vi "DisplayText.vi"(10 "text":string, 11 "Grid":T1) -> (3 "new picture":picture)   [LabVIEW 2020]
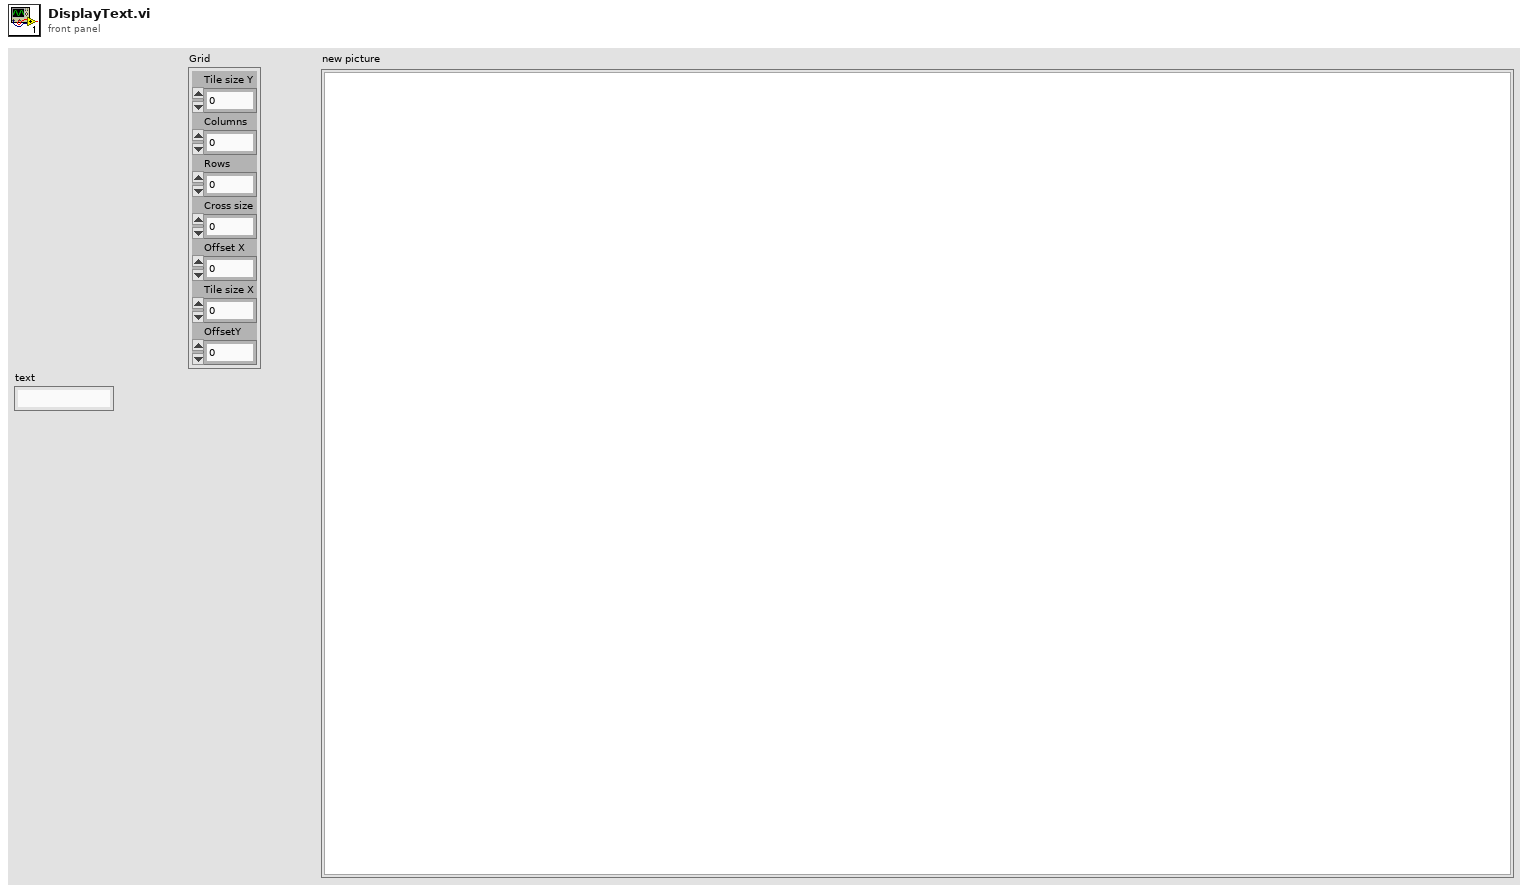
[diagram p1: front panel]
types:
  T1 = cluster{"Tile size Y":dbl, "Columns":dbl, "Rows":dbl, "Cross size":dbl, "Offset X":dbl, "Tile size X":dbl, "OffsetY":dbl}
  T2 = enum16{"User-specified Font", "Application Font", "System Font", "Dialog Font"}
  T3 = cluster{"Font Name:":string, "Size":i16, "Strikeout?":bool, "Italic?":bool, "Underline?":bool, "Outline?":bool, "Shadow?":bool, "Bold?":bool}
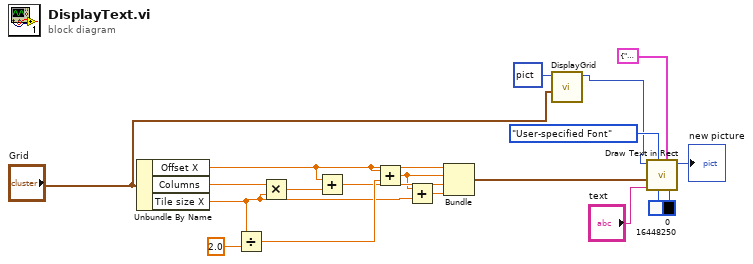
[diagram p0: block diagram]
diagram:
  n1 = Unbundle By Name("Grid") -> ("Offset X"=w9:dbl, "Columns"=w10:dbl, "Tile size X"=w5:dbl)
  n2 = Divide(x=w5, y=2.0) -> (x/y=w11:dbl)
  n3 = Multiply(x=w10, y=w5) -> (x*y=w8:dbl)
  n4 = Add(x=w9, y=w8) -> (x+y=w7:dbl)
  n5 = Add(x=w9, y=w11) -> (x+y=w4:dbl)
  n6 = Add(x=w4, y=w5) -> (x+y=w6:dbl)
  n7 = Bundle("Offset X"=w9, w4, w7, w6) -> (w19:cluster{"Offset X":dbl, dbl, dbl, dbl})  [unwired: 1 in]
  n8 = call "DisplayGrid.vi"("Grid"="Grid", "input picture"=picture data[5B]) -> ("new picture"=w3:picture)  [unwired: 9 in]
  n9 = call <vilib>:"Draw Text in Rect.vi"("BG color(transparent)"=u32 0 ("text color(black)"), "[user-specified font]"=T3 {"Font Name:"="Normal", "Size"=50, "Strikeout?"=FALSE, "Italic?"=FALSE, "Underline?"=FALSE, "Outline?"=FALSE, "Shadow?"=FALSE, "Bold?"=TRUE}, "text color(black)"=u32 16448250, "desired font(Application)"=T2."User-specified Font", "text"="text", "rect"=w19, "picture"=w3) -> ("new picture"=→"new picture":picture)  [unwired: 4 in]
